vi "releasePressureOld.vi"(7 "LabVIEW Web Service Request":refnum<class "Web Request.lvclass">, 9 "targetPressure":dbl, 10 "maximumTolerance":dbl, 11 "minimumTolerance":dbl) -> (2 "current pr":dbl, 3 "maximumPressure":dbl format="%0.2f")   [LabVIEW 2015]
uses:
  Control test 1.ctl
  <vilib>/wsapi/Web Request.lvclass
  <vilib>/Waveform/WDTOps.llb/WDT Append Waveforms DBL.vi
panel:
  in  "Start":bool
  in  "stop (F)":bool
  out "data":T1
  out "value":string
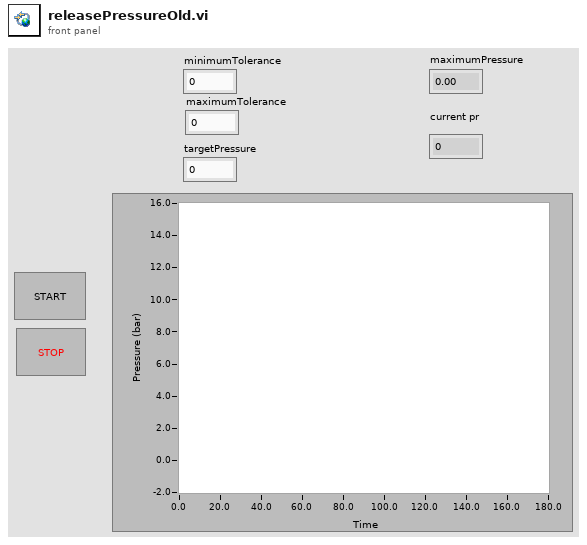
[diagram p1: front panel]
types:
  T1 = typedef "Control test 1.ctl" = dynamicdata
  T2 = typedef "imagedata.ctl" = cluster{"image type":i32, "image depth":i32, "image":u8[], "mask":u8[], "colors":u32[], "Rectangle":cluster{"left":i16, "top":i16, "right":i16, "bottom":i16}}
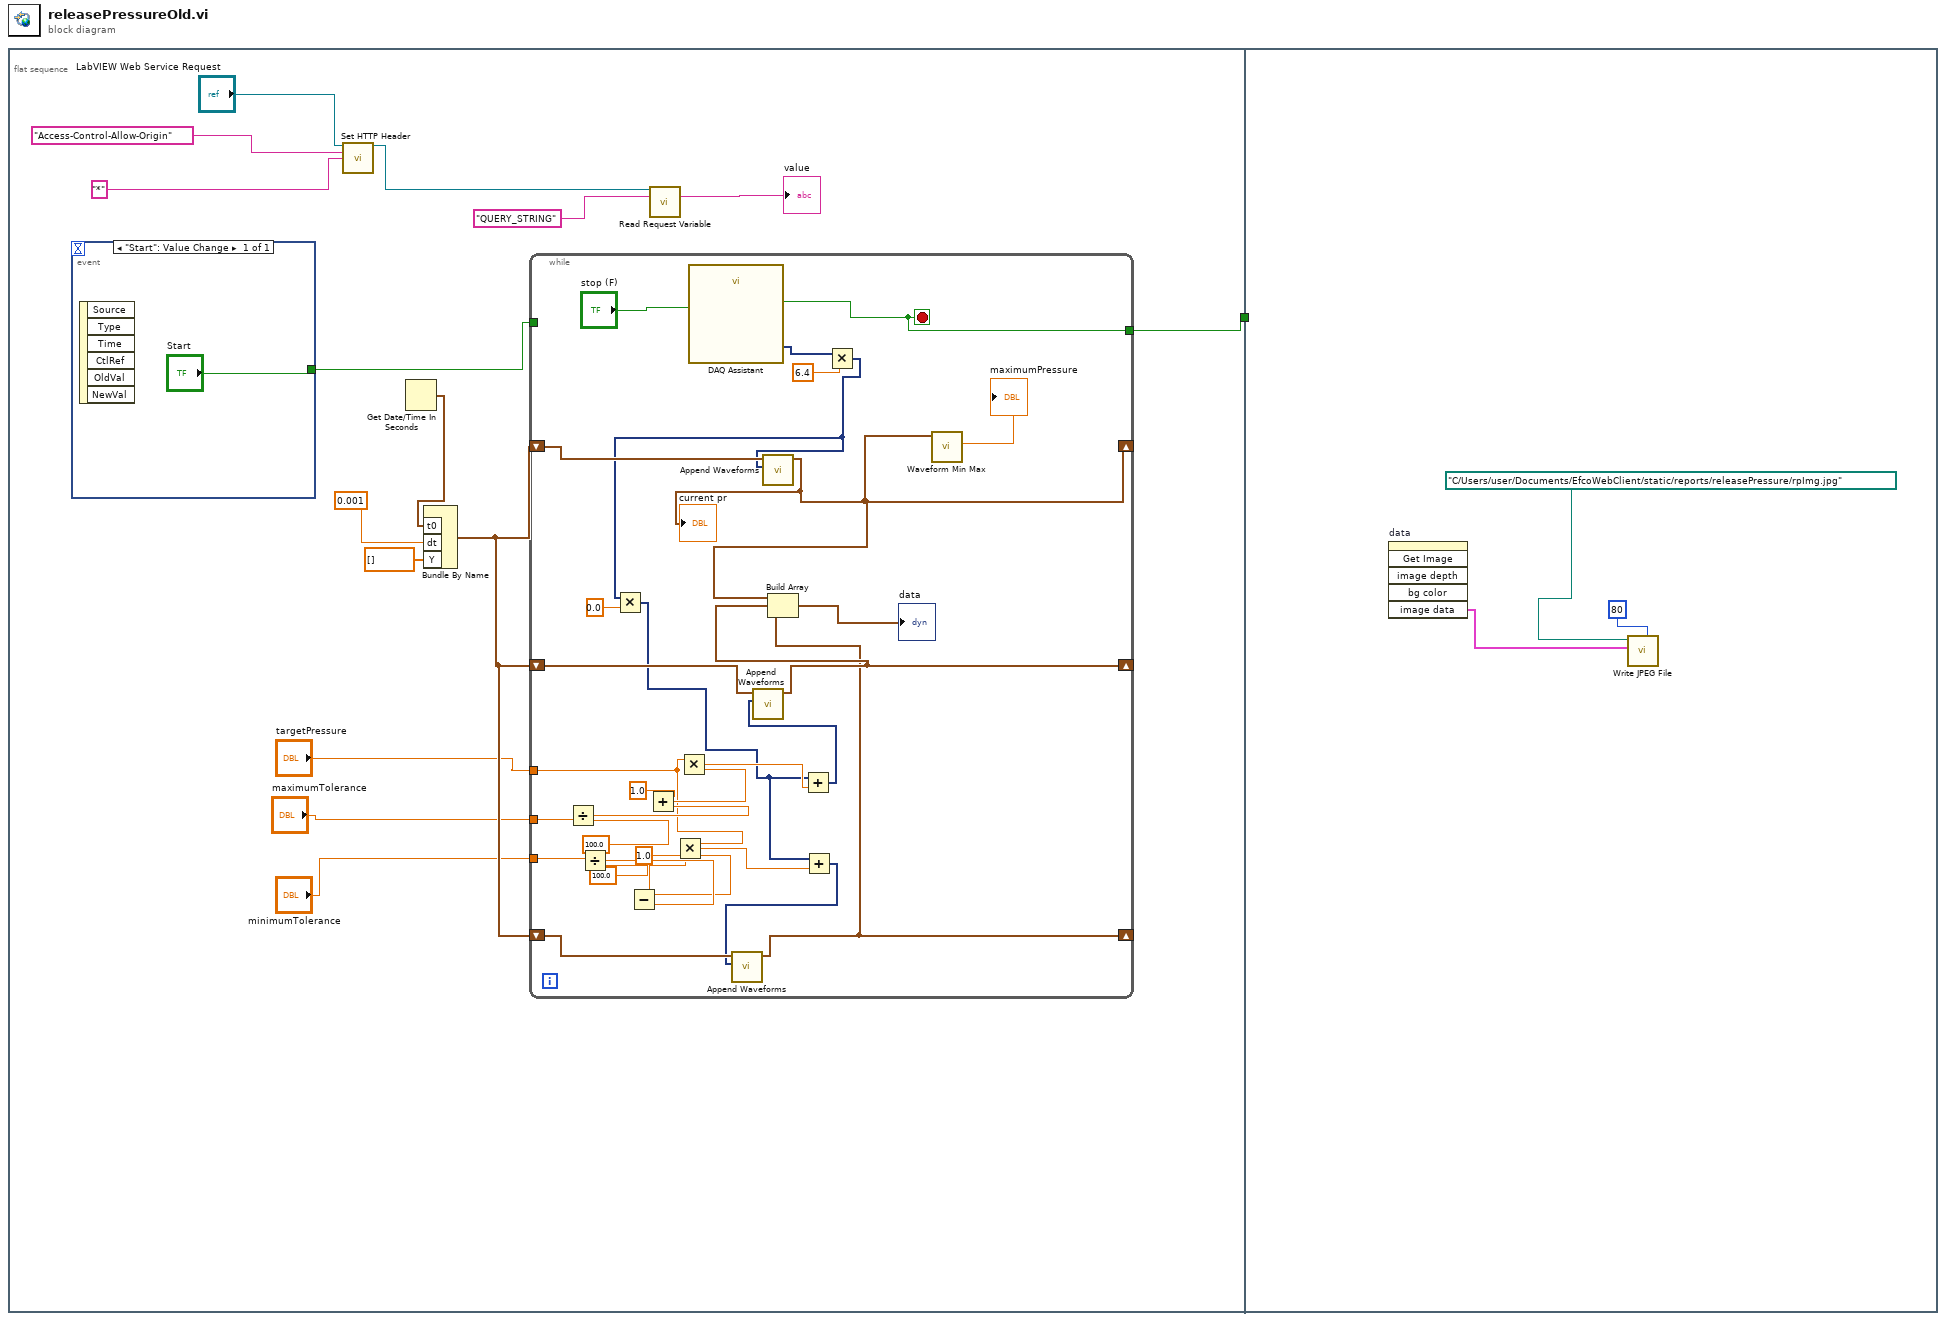
[diagram p0: block diagram]
diagram:
  n1 = flat-sequence {
    tunnel: [w3] -> w1
    tunnel: w1 -> [_]
    frame #0 {
      n2 = event shown="[0] \"Start\": Value Change" {
        selector: _ -> [_]
        dyn-events: _ -> [_]
        timeout: _ -> [_]
        tunnel: ["Start"] -> w2
        event "Start": Value Change {
          n3 = event-data() -> ()  [unwired: 1 in, 6 out]
        }
      }
      n4 = call <vilib>:"Set HTTP Header.vi"("LabVIEW Web Service Request"="LabVIEW Web Service Request", "header"="Access-Control-Allow-Origin", "header value"="*") -> ("LabVIEW Web Service Request out"=w6:refnum<class "Web Request.lvclass">)  [unwired: 11 in, 1 out]
      n5 = Get Date/Time In Seconds() -> (seconds since 1Jan1904=w13:timestamp)
      n6 = Bundle By Name("t0"=w13, "dt"=0.001, "Y"=dbl[] []) -> (w12:waveform(dbl))  [unwired: 1 in]
      n7 = while {
        shift-right: [w21] -> _
        shift-left: w12 -> [w24]
        shift-right: [w44] -> _
        shift-left: w12 -> [w45]
        tunnel: "maximumTolerance" -> [w43]
        tunnel: "minimumTolerance" -> [w41]
        tunnel: "targetPressure" -> [w33]
        shift-right: [w20] -> _
        shift-left: w12 -> [w29]
        tunnel: [w18] -> w3
        tunnel: w2 -> [_]
        stop <- w18 stop-if-true
        n8 = Divide(x=w43, y=100.0) -> (x/y=w38:dbl)
        n9 = Divide(x=w41, y=100.0) -> (x/y=w37:dbl)
        n10 = Subtract(x=1.0, y=w37) -> (x-y=w35:dbl)
        n11 = Add(x=1.0, y=w38) -> (x+y=w34:dbl)
        n12 = Multiply(x=w33, y=w35) -> (x*y=w27:dbl)
        n13 = Multiply(x=w33, y=w34) -> (x*y=w31:dbl)
        n14 = call "DAQ Assistant"("stop (F)"="stop (F)") -> ("data"=w25:dynamicdata, "stopped"=w18:bool)  [unwired: 15 in, 2 out]
        n15 = Multiply(x=w25, y=6.4) -> (x*y=w22:dynamicdata)
        n16 = Multiply(x=w22, y=0.0) -> (x*y=w28:dynamicdata)
        n17 = call-poly <vilib>:"Append Waveforms.vi"("waveform B"=w22, "waveform A"=w24) -> ("waveform out"=w21:waveform(dbl))  [unwired: 8 in, 1 out]
        "current pr" <- w21
        n18 = Add(x=w28, y=w31) -> (x+y=w30:dynamicdata)
        n19 = call-poly <vilib>:"Append Waveforms.vi"("waveform B"=w30, "waveform A"=w45) -> ("waveform out"=w44:waveform(dbl))  [unwired: 8 in, 1 out]
        n20 = Add(x=w28, y=w27) -> (x+y=w26:dynamicdata)
        n21 = call-poly <vilib>:"Append Waveforms.vi"("waveform B"=w26, "waveform A"=w29) -> ("waveform out"=w20:waveform(dbl))  [unwired: 8 in, 1 out]
        n22 = Build Array(w21, w44, w20) -> (→"data":waveform(dbl)[])
        n23 = call <vilib>:"Waveform Min Max.vi"("waveform in"=w21) -> ("Y max"=→"maximumPressure":dbl)  [unwired: 5 in, 5 out]
      }
      n24 = call <vilib>:"Read Request Variable.vi"("LabVIEW Web Service Request"=w6, "variable name"="QUERY_STRING") -> ("value"=→"value":string)  [unwired: 11 in, 2 out]
    }
    frame #1 {
      n25 = invoke on="data" class="WFGraph (strict)" method="Get Image"() -> ("image data"=w50:T2)  [unwired: 6 in, 5 out]
      n26 = call <vilib>:"Write JPEG File.vi"("quality (80)"=80, "image data"=w50, "path to JPEG file"=path "C:/Users/user/Documents/EfcoWebClient/static/reports/releasePressure/rpImg.jpg") -> ()  [unwired: 7 in, 2 out]
    }
  }
